vi "HW2_pt10 (1).vi"() -> ()   [LabVIEW 2021]
panel:
  out "Num_3_Presses":dbl
  out "Num_r_Presses":dbl
  out "turn":dbl
  out "Vref":dbl
  out "Num_q_Presses":dbl
  out "Key Pressed":i16
  out "Y":dbl
  out "X":dbl
  out "RecValue3":dbl
  out "RecValue4":dbl
  out "RecValue5":dbl
  out "RecValue6":dbl
  out "RecValue 7":dbl
  out "RecValue8":dbl
  in  "Size of Rectangle":i16=20
  in  "Display History":bool
  out "2D picture":picture
  in  "SendValue 8":dbl
  in  "SendValue 7":dbl
  in  "SendValue 6":dbl
  in  "SendValue 5":dbl
  in  "SendValue 4":dbl
  in  "SendValue 3":dbl
  in  "turn":dbl
  in  "Vref":dbl
  in  "Send Button":bool
  in  "stop":bool
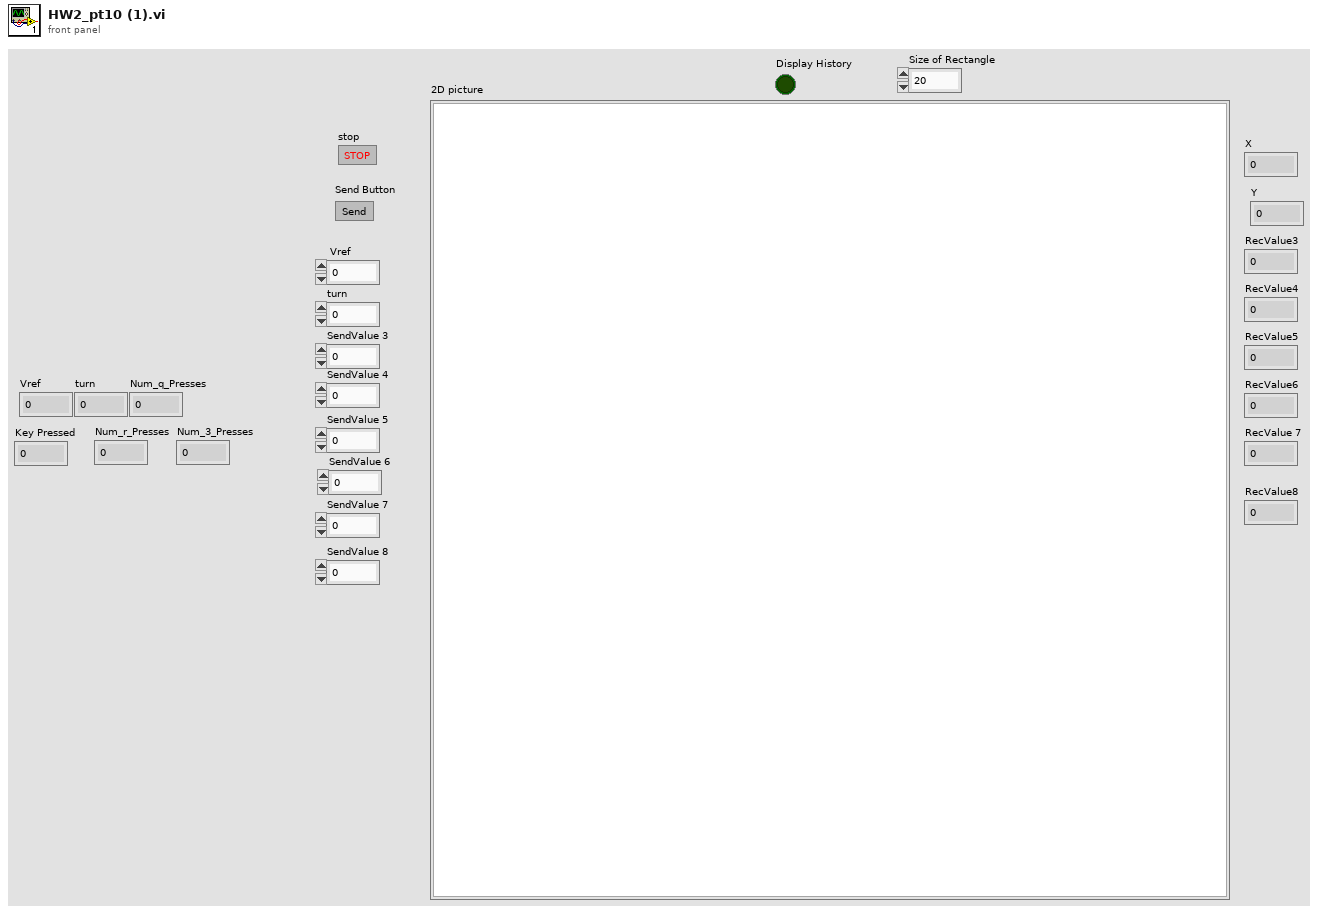
[diagram p1: front panel]
types:
  T1 = enum16{"Standard", "Buffered", "CRLF", "Immediate"}
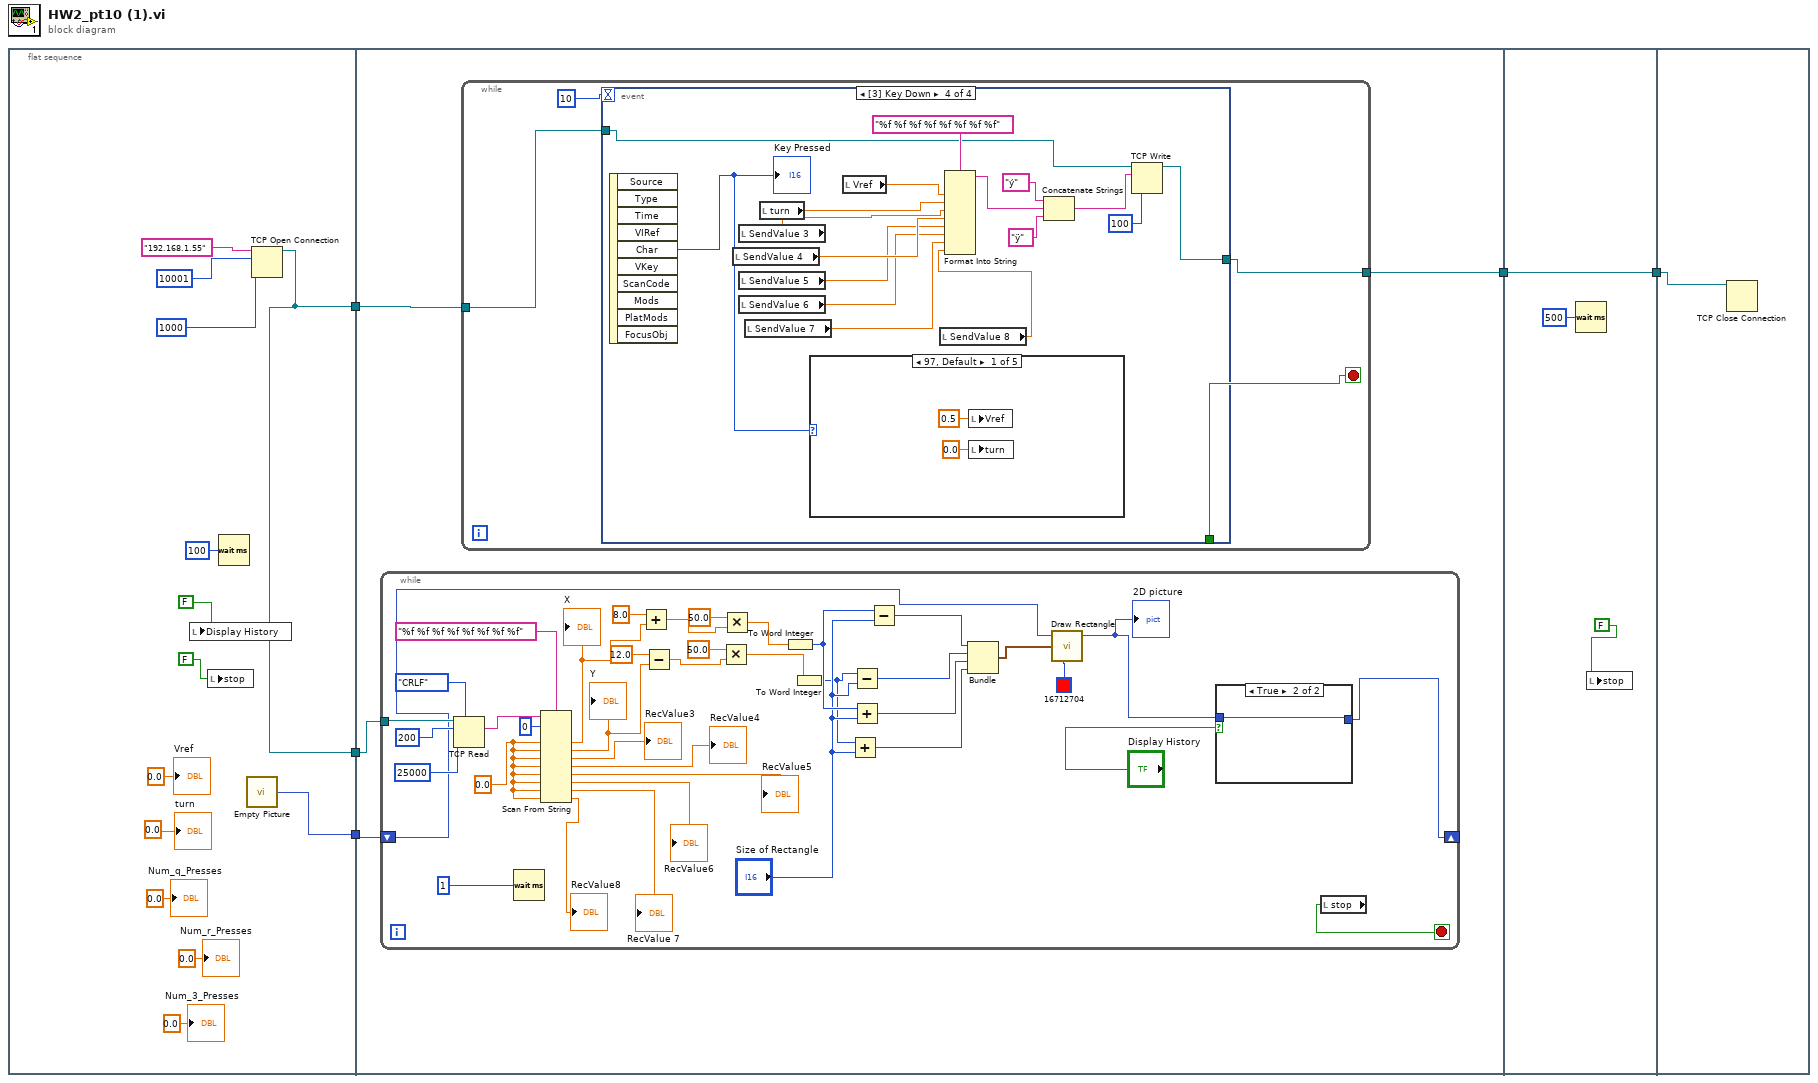
[diagram p0: block diagram]
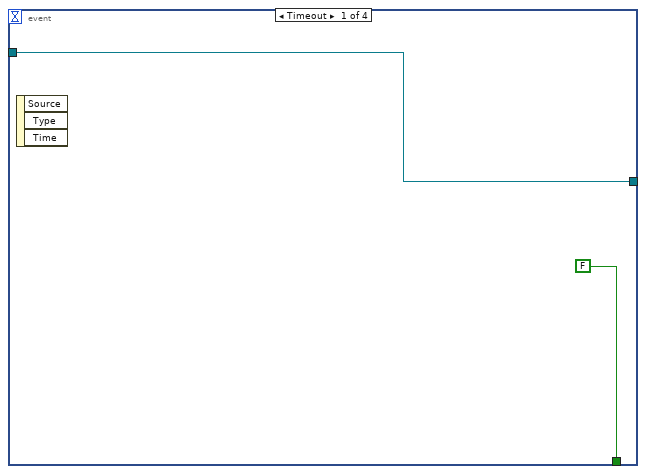
[diagram p2: hidden frame]
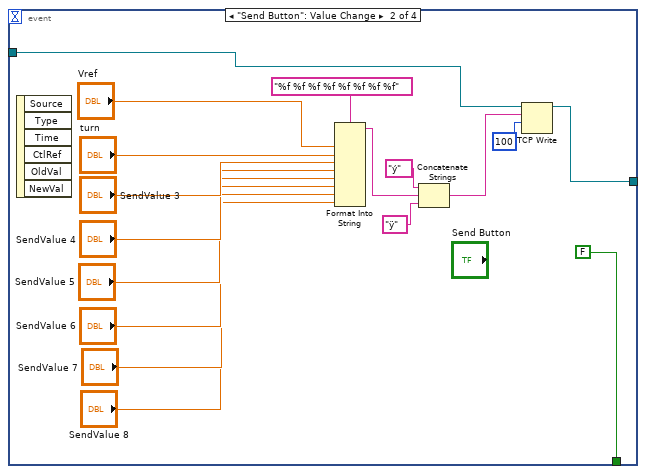
[diagram p3: hidden frame]
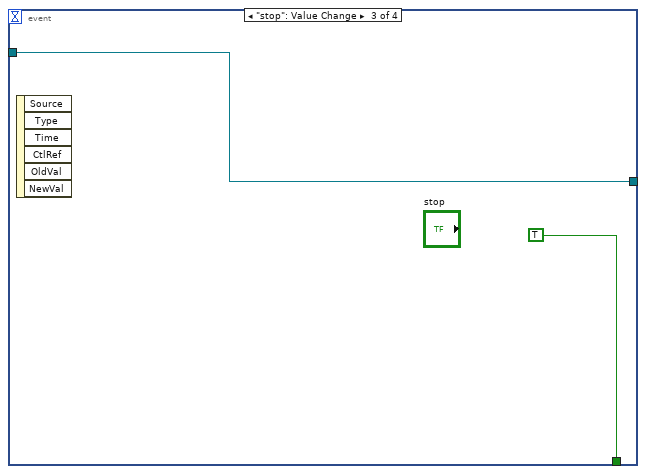
[diagram p4: hidden frame]
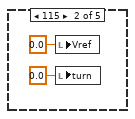
[diagram p5: hidden frame]
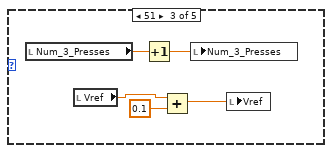
[diagram p6: hidden frame]
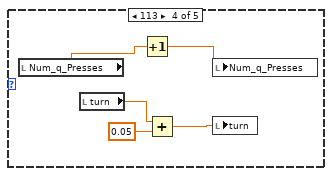
[diagram p7: hidden frame]
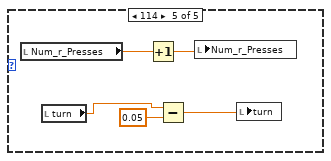
[diagram p8: hidden frame]
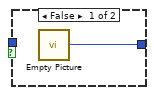
[diagram p9: hidden frame]
diagram:
  n1 = flat-sequence {
    tunnel: [w11] -> w5
    tunnel: [w12] -> w2
    tunnel: [w11] -> w1
    tunnel: w5 -> [w22]
    tunnel: [w21] -> w3
    tunnel: w2 -> [w19]
    tunnel: w1 -> [w20]
    tunnel: [w126] -> w4
    tunnel: w3 -> [w126]
    tunnel: w4 -> [w128]
    frame #0 {
      n2 = local write "Display History"(FALSE) -> ()
      n3 = local write "stop"(FALSE) -> ()
      n4 = Wait (ms)(milliseconds to wait=u32 100) -> ()  [unwired: 1 out]
      n5 = call "Empty Picture"() -> ("empty picture"=w12:picture)
      n6 = TCP Open Connection(address="192.168.1.55", remote port or service name=u16 10001, timeout ms (60000)=1000) -> (connection ID=w11:refnum<k5>)  [unwired: 2 in, 1 out]
      "Num_q_Presses" <- 0.0 ("Num_q_Presses 2")
      "Vref" <- 0.0
      "turn" <- 0.0
      "Num_r_Presses" <- 0.0 ("Num_q_Presses 2")
      "Num_3_Presses" <- 0.0 ("Num_q_Presses 2")
    }
    frame #1 {
      n7 = while {
        tunnel: w20 -> [w108]
        shift-right: [w84] -> _
        shift-left: w19 -> [w85]
        stop <- w86 stop-if-true
        w101 = 0.0
        n8 = TCP Read(connection ID=w108, bytes to read=200, 7:T1."CRLF" ("mode (standard)"), 9:25000 ("timeout ms (25000)")) -> (data out=w104:string)  [unwired: 1 in, 2 out]
        n9 = Wait (ms)(milliseconds to wait=u32 1) -> ()  [unwired: 1 out]
        n10 = Scan From String(format string="%f %f %f %f %f %f %f %f", input string=w104, initial scan location=u32 0, default 1=w101, default 2=w101, default 3=w101, default 4=w101, default 5=w101, default 6=w101, default 7=w101, default 8=w101) -> (output 1=w88:dbl, output 2=w87:dbl, output 3=→"RecValue3":dbl, output 4=→"RecValue4":dbl, output 5=→"RecValue5":dbl, output 6=→"RecValue6":dbl, output 7=→"RecValue 7":dbl, output 8=→"RecValue8":dbl)  [unwired: 1 in, 3 out]
        "X" <- w88
        "Y" <- w87
        n11 = Add(x=8.0, y=w88) -> (x+y=w92:dbl)
        n12 = Subtract(x=12.0, y=w87) -> (x-y=w91:dbl)
        n13 = Multiply(x=50.0, y=w91) -> (x*y=w118:dbl)
        n14 = Multiply(x=50.0, y=w92) -> (x*y=w117:dbl)
        n15 = To Word Integer(number=w117) -> (16bit integer=w116:i16)
        n16 = To Word Integer(number=w118) -> (16bit integer=w114:i16)
        n17 = Add(x=w114, y="Size of Rectangle") -> (x+y=w113:i16)
        n18 = Subtract(x=w114, y="Size of Rectangle") -> (x-y=w111:i16)
        n19 = Add(x=w116, y="Size of Rectangle") -> (x+y=w112:i16)
        n20 = Subtract(x=w116, y="Size of Rectangle") -> (x-y=w110:i16)
        n21 = Bundle(w110, w111, w112, w113) -> (w119:cluster{i16, i16, i16, i16})  [unwired: 1 in]
        n22 = call <vilib>:"Draw Rectangle.vi"("picture"=w85, "rect"=w119, "color(black)"=u32 16712704) -> ("new picture"=w120:picture)  [unwired: 6 in]
        "2D picture" <- w120
        n23 = case shown="True" "Display History" {
          tunnel: [w123 w124] -> w84
          tunnel: w120 -> [_ w124]
          frame False {
            n24 = call "Empty Picture"() -> ("empty picture"=w123:picture)
          }
          frame True {
          }
        }
        n25 = local read "stop"() -> (w86:bool)
      }
      n26 = while {
        tunnel: w22 -> [w24]
        tunnel: [w23] -> w21
        stop <- w25 stop-if-true
        n27 = event shown="[3] Key Down" {
          selector: _ -> [_ _ _ _]
          dyn-events: _ -> [_ _ _ _]
          timeout: 10 -> [_ _ _ _]
          tunnel: [FALSE FALSE ("stop") TRUE ("stop") _] -> w25
          tunnel: [w27 w29 w47 w48] -> w23
          tunnel: w24 -> [w27 w30 w47 w49]
          event Timeout {
            n28 = event-data() -> ()  [unwired: 1 in, 3 out]
          }
          event "Send Button": Value Change {
            n29 = event-data() -> ()  [unwired: 1 in, 6 out]
            n30 = Format Into String(format string="%f %f %f %f %f %f %f %f", "Vref", "turn", "SendValue 3", "SendValue 4", "SendValue 5", "SendValue 6", "SendValue 7", "SendValue 8") -> (resulting string=w40:string)  [unwired: 2 in, 1 out]
            n31 = Concatenate Strings("ý" ("string"), w40, "ÿ" ("string")) -> (w41:string)
            n32 = TCP Write(connection ID=w30, data in=w41, 9:100 ("timeout ms (25000)")) -> (connection ID out=w29:refnum<k5>)  [unwired: 1 in, 2 out]
          }
          event "stop": Value Change {
            n33 = event-data() -> ()  [unwired: 1 in, 6 out]
          }
          event Key Down {
            n34 = event-data() -> ("Char"=w64:i16)  [unwired: 1 in, 9 out]
            "Key Pressed" <- w64
            n35 = local read "SendValue 4"() -> (w59:dbl)
            n36 = local read "SendValue 3"() -> (w60:dbl)
            n37 = local read "SendValue 5"() -> (w58:dbl)
            n38 = local read "SendValue 6"() -> (w57:dbl)
            n39 = local read "SendValue 7"() -> (w56:dbl)
            n40 = local read "turn"() -> (w61:dbl)
            n41 = case shown="97, Default" w64 {
              frame 97, Default {
                n42 = local write "Vref"(0.5 ("Vref")) -> ()
                n43 = local write "turn"(0.0 ("turn")) -> ()
              }
              frame 115 {
                n44 = local write "Vref"(0.0 ("Vref")) -> ()
                n45 = local write "turn"(0.0 ("turn")) -> ()
              }
              frame 51 {
                n46 = local read "Num_3_Presses"() -> (w70:dbl)
                n47 = local read "Vref"() -> (w72:dbl)
                n48 = Increment(x=w70) -> (x+1=w69:dbl)
                n49 = Add(x=w72, y=0.1) -> (x+y=w71:dbl)
                n50 = local write "Num_3_Presses"(w69) -> ()
                n51 = local write "Vref"(w71) -> ()
              }
              frame 113 {
                n52 = local read "Num_q_Presses"() -> (w78:dbl)
                n53 = local read "turn"() -> (w75:dbl)
                n54 = Increment(x=w78) -> (x+1=w77:dbl)
                n55 = Add(x=w75, y=0.05) -> (x+y=w74:dbl)
                n56 = local write "Num_q_Presses"(w77) -> ()
                n57 = local write "turn"(w74) -> ()
              }
              frame 114 {
                n58 = local read "Num_r_Presses"() -> (w80:dbl)
                n59 = local read "turn"() -> (w82:dbl)
                n60 = Increment(x=w80) -> (x+1=w79:dbl)
                n61 = Subtract(x=w82, y=0.05) -> (x-y=w81:dbl)
                n62 = local write "Num_r_Presses"(w79) -> ()
                n63 = local write "turn"(w81) -> ()
              }
            }
            n64 = local read "Vref"() -> (w62:dbl)
            n65 = local read "SendValue 8"() -> (w55:dbl)
            n66 = Format Into String(format string="%f %f %f %f %f %f %f %f", w62, w61, w60, w59, w58, w57, w56, w55) -> (resulting string=w52:string)  [unwired: 2 in, 1 out]
            n67 = Concatenate Strings("ý" ("string"), w52, "ÿ" ("string")) -> (w50:string)
            n68 = TCP Write(connection ID=w49, data in=w50, 9:100 ("timeout ms (25000)")) -> (connection ID out=w48:refnum<k5>)  [unwired: 1 in, 2 out]
          }
        }
      }
    }
    frame #2 {
      n69 = Wait (ms)(milliseconds to wait=u32 500) -> ()  [unwired: 1 out]
      n70 = local write "stop"(FALSE) -> ()
    }
    frame #3 {
      n71 = TCP Close Connection(connection ID=w128) -> ()  [unwired: 2 in, 2 out]
    }
  }
